vi "test Add Multiple Custom Devices.vi"(8 "error in":errorcluster, 11 "TestCase in":refnum<class "Scripting.lvclass">) -> (0 "error out":errorcluster, 3 "TestCase out":refnum<class "Scripting.lvclass">)   [LabVIEW 2020, in "Scripting.lvclass"]
uses:
  Scripting.lvclass
  C:/dev/git/niveristand-custom-device-testing-tools/VeriStandScriptingTestCase/VeriStandScriptingTestCase.lvclass
  niveristand-custom-device-testing-tools/VeriStandScriptingTestCase/VeriStandScriptingTestCase.lvclass/VeriStandScriptingTestCase.ctl
  niveristand-custom-device-testing-tools/VeriStandScriptingTestCase/Read Target.vi
  NationalInstruments.VeriStand.SystemDefinitionAPI
  <vilib>/addons/_JKI Toolkits/VI Tester/TestCase.llb/TestCase.lvclass
  Scripting/AIM MIL-STD-1553 Scripting.lvlib
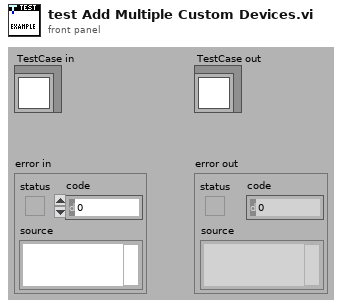
[diagram p1: front panel]
types:
  T1 = typedef "Custom Device API.lvlib/Custom Device Item Ref.ctl" = u64
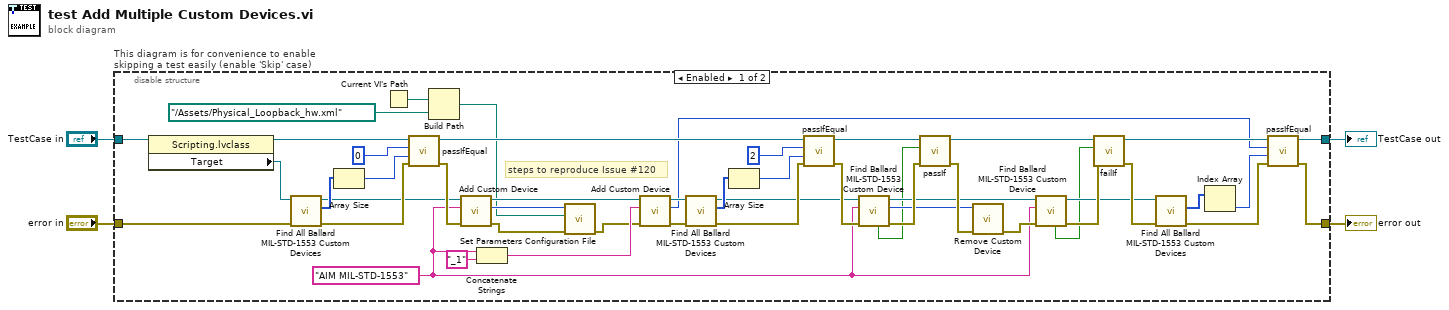
[diagram p0: block diagram]
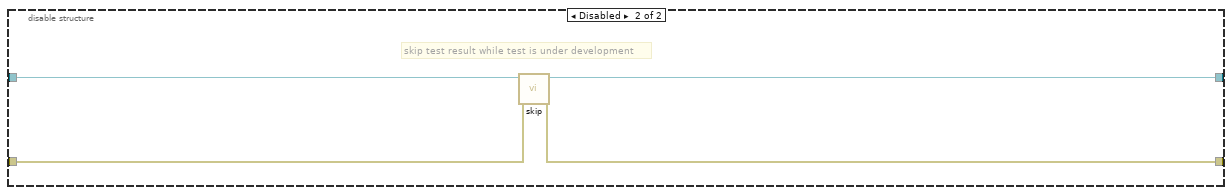
[diagram p2: hidden frame]
diagram:
  n1 = disable-structure "This diagram is for convenience to enable skipping a test easily (enable 'Skip' case)" shown="Enabled" {
    disable-tunnel: "TestCase in" -> [w19 w56]
    disable-tunnel: [w21 w54] -> w1
    disable-tunnel: [w20 w55] -> w3
    disable-tunnel: "error in" -> [w52 w53]
    frame Enabled {
      w29 = "AIM MIL-STD-1553" ("name")
      # "steps to reproduce Issue #120"
      n2 = property class="Scripting.lvclass"(reference=w19) -> (reference out=w17:refnum<class "Scripting.lvclass">, "Target"=w18:refnum<k24>)  [unwired: 1 in, 1 out]
      n3 = call "Find All Ballard MIL-STD-1553 Custom Devices.vi"("error in"=w52, "target in"=w18) -> ("error out"=w48:errorcluster, "Ballard MIL-STD-1553 custom devices"=w51:T1[], "target out"=w46:refnum<k24>)  [unwired: 7 in]
      n4 = Array Size(array=w51) -> (size(s)=w50:i32)
      n5 = Current VI's Path() -> (path=w13:path)
      n6 = call-dynamic "passIfEqual.vi"("error in (no error)"=w48, "y"=w50, "x"=0 ("size(s)"), "TestCase in"=w17) -> ("error out"=w47:errorcluster, "TestCase out"=w16:refnum<class "Scripting.lvclass">)  [unwired: 6 in]
      n7 = Build Path(base path=w13, name or relative path=path "../Assets/Physical_Loopback_hw.xml") -> (appended path=w10:path)
      n8 = call "Add Custom Device.vi"("error in"=w47, "name"=w29, "target in"=w46) -> ("error out"=w14:errorcluster, "Ballard MIL-STD 1553 custom device"=w15:T1, "target out"=w44:refnum<k24>)  [unwired: 6 in]
      n9 = Concatenate Strings(w29, "_1" ("string")) -> (w43:string)
      n10 = call "Set Parameters Configuration File.vi"("error in"=w14, "parameters configuration file path"=w10, "Ballard MIL-STD 1553 custom device in"=w15) -> ("error out"=w11:errorcluster)  [unwired: 7 in, 1 out]
      n11 = call "Add Custom Device.vi"("error in"=w11, "name"=w43, "target in"=w44) -> ("error out"=w42:errorcluster, "Ballard MIL-STD 1553 custom device"=w5:T1, "target out"=w41:refnum<k24>)  [unwired: 6 in]
      n12 = call "Find All Ballard MIL-STD-1553 Custom Devices.vi"("error in"=w42, "target in"=w41) -> ("error out"=w37:errorcluster, "Ballard MIL-STD-1553 custom devices"=w38:T1[], "target out"=w35:refnum<k24>)  [unwired: 7 in]
      n13 = Array Size(array=w38) -> (size(s)=w39:i32)
      n14 = call-dynamic "passIfEqual.vi"("error in (no error)"=w37, "y"=w39, "x"=2 ("size(s)"), "TestCase in"=w16) -> ("error out"=w36:errorcluster, "TestCase out"=w34:refnum<class "Scripting.lvclass">)  [unwired: 6 in]
      n15 = call "Find Ballard MIL-STD-1553 Custom Device.vi"("error in"=w36, "name"=w29, "target in"=w35) -> ("error out"=w33:errorcluster, "Ballard MIL-STD 1553 custom device"=w31:T1, "target out"=w28:refnum<k24>, "found?"=w9:bool)  [unwired: 5 in]
      n16 = call-dynamic "passIf.vi"("error in (no error)"=w33, "pass"=w9, "TestCase in"=w34) -> ("error out"=w32:errorcluster, "TestCase out"=w27:refnum<class "Scripting.lvclass">)  [unwired: 7 in]
      n17 = call "Remove Custom Device.vi"("error in"=w32, "Ballard MIL-STD 1553 custom device"=w31) -> ("error out"=w30:errorcluster)  [unwired: 9 in]
      n18 = call "Find Ballard MIL-STD-1553 Custom Device.vi"("error in"=w30, "name"=w29, "target in"=w28) -> ("error out"=w26:errorcluster, "target out"=w24:refnum<k24>, "found?"=w8:bool)  [unwired: 5 in, 1 out]
      n19 = call-dynamic "failIf.vi"("error in (no error)"=w26, "fail"=w8, "TestCase in"=w27) -> ("error out"=w25:errorcluster, "TestCase out"=w23:refnum<class "Scripting.lvclass">)  [unwired: 7 in]
      n20 = call "Find All Ballard MIL-STD-1553 Custom Devices.vi"("error in"=w25, "target in"=w24) -> ("error out"=w22:errorcluster, "Ballard MIL-STD-1553 custom devices"=w7:T1[])  [unwired: 7 in, 1 out]
      n21 = Index Array(array=w7) -> (element=w6:T1)  [unwired: 1 in]
      n22 = call-dynamic "passIfEqual.vi"("error in (no error)"=w22, "y"=w6, "x"=w5, "TestCase in"=w23) -> ("error out"=w20:errorcluster, "TestCase out"=w21:refnum<class "Scripting.lvclass">)  [unwired: 6 in]
    }
    frame Disabled {
      # "skip test result while test is under development"
      n23 = call <vilib>:"skip.vi"("error in (no error)"=w53, "TestCase in"=w56) -> ("error out"=w55:errorcluster, "TestCase out"=w54:refnum<class "Scripting.lvclass">)  [unwired: 8 in]
    }
  }
  "error out" <- w3
  "TestCase out" <- w1
